vi "Lab1_A3_subVI.vi"(7 "Amplitude":dbl, 8 "Time":dbl, 9 "Frequency":dbl, 10 "Signal Type":dbl) -> (3 "Signal":dbl)   [LabVIEW 2020]
uses:
  <vilib>/ptbypt/NI_PtbyPt.lvlib
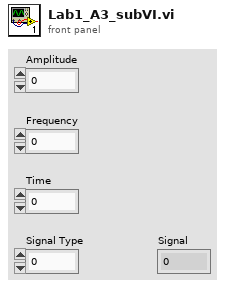
[diagram p1: front panel]
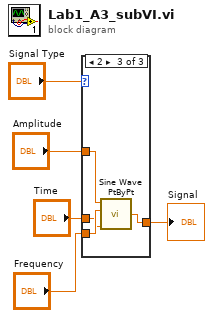
[diagram p0: block diagram]
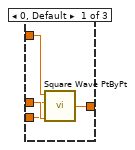
[diagram p2: hidden frame]
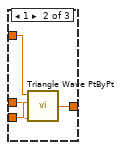
[diagram p3: hidden frame]
diagram:
  n1 = case shown="2" "Signal Type" {
    tunnel: "Frequency" -> [w6 w11 w16]
    tunnel: "Time" -> [w7 w10 w14]
    tunnel: "Amplitude" -> [w8 w13 w17]
    tunnel: [w9 w12 w15] -> w2
    frame 0, Default {
      n2 = call <vilib>:"Square Wave PtByPt.vi"("amplitude"=w8, "frequency"=w6, "time"=w7) -> ("square wave"=w9:dbl)  [unwired: 2 in]
    }
    frame 1 {
      n3 = call <vilib>:"Triangle Wave PtByPt.vi"("time"=w10, "frequency"=w11, "amplitude"=w13) -> ("triangle wave"=w12:dbl)  [unwired: 1 in]
    }
    frame 2 {
      n4 = call <vilib>:"Sine Wave PtByPt.vi"("time"=w14, "frequency"=w16, "amplitude"=w17) -> ("sine wave"=w15:dbl)  [unwired: 1 in]
    }
  }
  "Signal" <- w2
